vi "Maruszak_Pracownia_6_global.vi"() -> ()   [LabVIEW 2019]
panel:
  in  "stop":bool
  out "Tablica bitów":bool[](array[boolean])
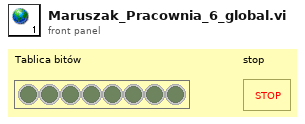
[diagram p1: front panel]
diagram:
